vi "获取存数据路径.vi"(11 "ModelEditInfo":T1={"AllModelFold"=path "", "AllModelNamePath"=path "", "所有零件型号"=[], "当前零件型号"="", "所有建立零件信息"=[], "当前零件序号"=0, "当前产品信息"={"产品型号"="J016-9STWH-A插头", "二维码拍照"=0, "Mark点拍照"=0}}) -> (3 "当天存数据路径":path)   [LabVIEW 2014]
uses:
  ModelEditSubVIs/ModeEditeControl.ctl
  ModelEditSubVIs/ModelInfo.ctl
  Global.vi
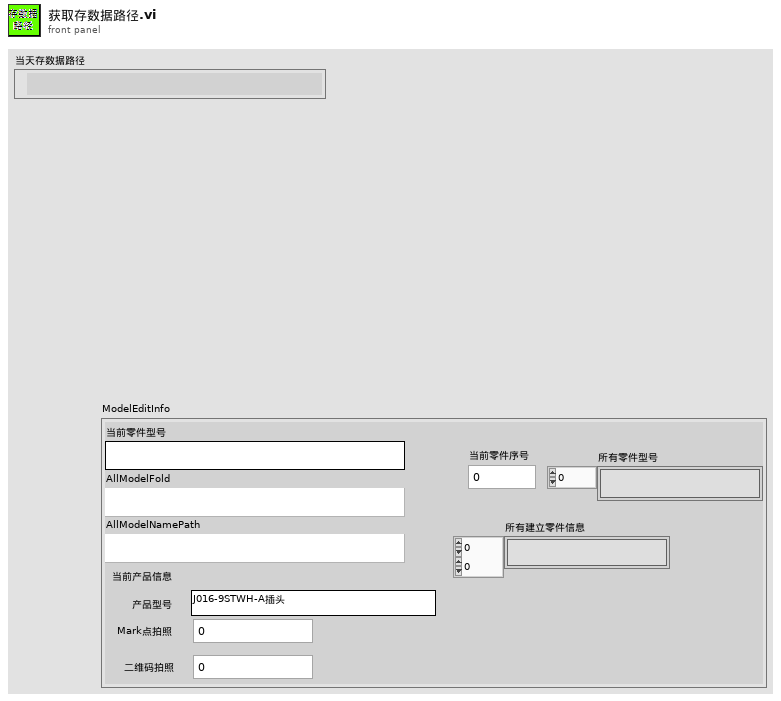
[diagram p1: front panel]
types:
  T1 = typedef "ModeEditeControl.ctl" = cluster{"AllModelFold":path, "AllModelNamePath":path, "所有零件型号":string[], "当前零件型号":string, "所有建立零件信息":string[][], "当前零件序号":i32, "当前产品信息":T2}
  T2 = typedef "ModelInfo.ctl" = cluster{"产品型号":string, "二维码拍照":u32, "Mark点拍照":u32}
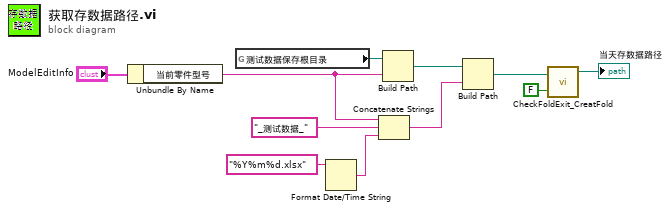
[diagram p0: block diagram]
diagram:
  n1 = Unbundle By Name("ModelEditInfo") -> ("当前零件型号"=w1:string)
  n2 = global read "Global.vi" "测试数据保存根目录"() -> (w7:path)
  n3 = Format Date/Time String(time format string (%c)="%Y%m%d.xlsx" ("时间格式字符串(%c)")) -> (date/time string=w10:string)  [unwired: 2 in]
  n4 = Concatenate Strings(w1, "_测试数据_" ("名称或相对路径"), w10) -> (w11:string)
  n5 = Build Path(base path=w7, name or relative path=w1) -> (appended path=w8:path)
  n6 = Build Path(base path=w8, name or relative path=w11) -> (appended path=w5:path)
  n7 = call "CheckFoldExit_CreatFold.vi"("path in"=w5, "FoldOrFile¡H"=FALSE) -> ("File out"=→"当天存数据路径":path)  [unwired: 2 out]
